vi "SetConfig.vi"(8 "error in":errorcluster, 10 "S2Config":T1 {"EC_PTEST_DELTA_BASELINE" format="%#_g psi"; "EC_PTEST_SCALE_FACTOR" min=0.0 max=1.0 step=0.01; "ECZ3_POFF_STABLE" format="%#_g sec"; "EC_PSTABLE_WAIT" format="%#_g sec"; "EC_PTEST_TIMER" format="%#_g sec"; "ECLOP_TIMER" format="%#_g sec"}, 11 "Global":T2={"Report Folder Path"=path "", "PT1_MIN"=0.0, "PT1_MAX"=0.0, "VENT_PMAX"=0.0, "LOP_TARGET"=0.0, "LOP_RAMP"=0.0, "LOP_LEAK_MAX"=0.0, "HIP_TARGET"=0.0, "HIP_RAMP"=0.0, "HIP_MIN"=0.0, "HIP_MAX"=0.0, "BLEED_TIME"=0.0, "LOP_MAX"=0.0, "LOP_MIN"=0.0, "PT131Com"="COM5", "PT231Com"="COM6", "PT331Com"="COM7", "PT431Com"="COM8", "PT531Com"="COM9", "PT631Com"="COM10"} {"LOP_MIN" format="%#_g PSI"; "LOP_MAX" format="%#_g PSI"; "BLEED_TIME" format="%#_g Sec"; "HIP_MAX" format="%#_g PSI"; "HIP_MIN" format="%#_g PSI"; "HIP_RAMP" format="%#_g Sec"; "HIP_TARGET" format="%#_g PSI"; "LOP_LEAK_MAX" format="%#_g PSI"; "LOP_RAMP" format="%#_g Sec"; "LOP_TARGET" format="%#_g PSI"; "VENT_PMAX" format="%#_g PSI"; "PT1_MAX" format="%#_g PSI"; "PT1_MIN" format="%#_g PSI"}) -> (0 "error out":errorcluster)   [LabVIEW 2018, in "S2.lvclass"]
uses:
  S2.lvclass
  Controller/Public Controls/GlobalConfig.ctl
  Controller/Public Controls/S2Config.ctl
  Queue/Queue Data.ctl
  Queue/State.ctl
  Controller/GUI.lvclass
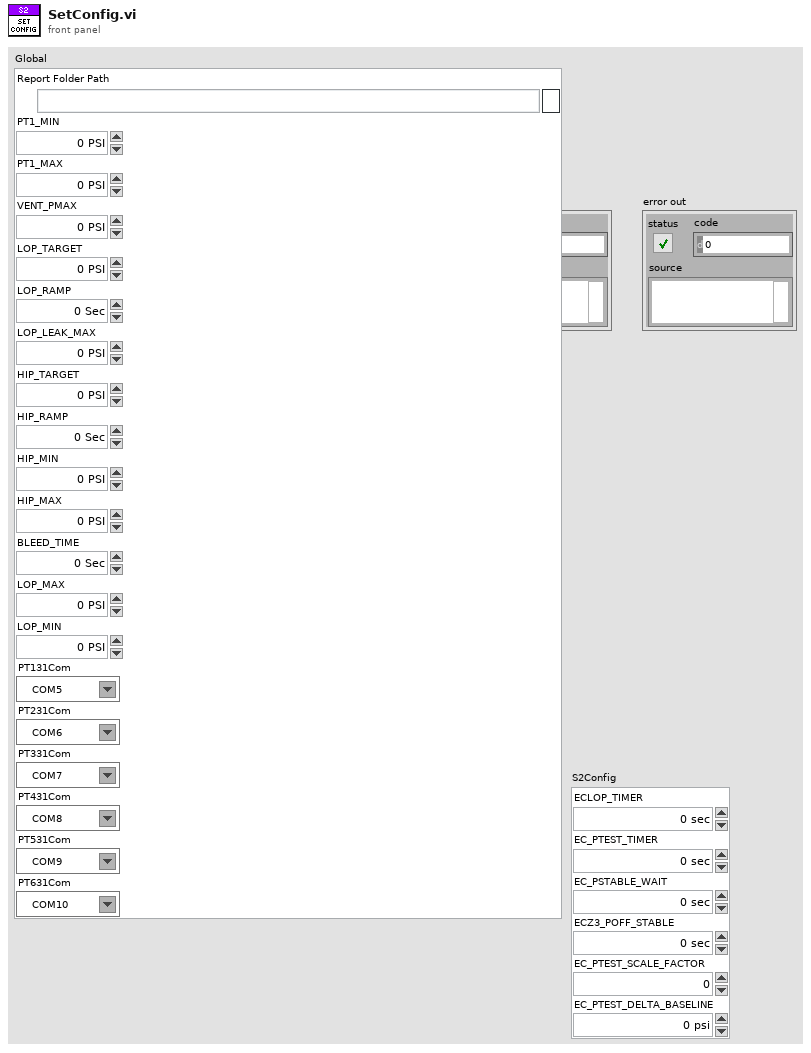
[diagram p1: front panel]
types:
  T1 = typedef "GUI.lvclass/S2Config.ctl" = cluster{"ECLOP_TIMER":dbl, "EC_PTEST_TIMER":dbl, "EC_PSTABLE_WAIT":dbl, "ECZ3_POFF_STABLE":dbl, "EC_PTEST_SCALE_FACTOR":dbl, "EC_PTEST_DELTA_BASELINE":dbl}
  T2 = typedef "GUI.lvclass/GlobalConfig.ctl" = cluster{"Report Folder Path":path, "PT1_MIN":dbl, "PT1_MAX":dbl, "VENT_PMAX":dbl, "LOP_TARGET":dbl, "LOP_RAMP":dbl, "LOP_LEAK_MAX":dbl, "HIP_TARGET":dbl, "HIP_RAMP":dbl, "HIP_MIN":dbl, "HIP_MAX":dbl, "BLEED_TIME":dbl, "LOP_MAX":dbl, "LOP_MIN":dbl, "PT131Com":refnum<visa-resource-name>, "PT231Com":refnum<visa-resource-name>, "PT331Com":refnum<visa-resource-name>, "PT431Com":refnum<visa-resource-name>, "PT531Com":refnum<visa-resource-name>, "PT631Com":refnum<visa-resource-name>}
  T3 = typedef "S2.lvclass/Queue Data.ctl" = cluster{"State":T4, "Data":variant}
  T4 = typedef "S2.lvclass/State.ctl" = enum16{"Initialize", "SetConfig", "AckAlarm", "Alarm", "Idle", "LockLid", "LowPressure", "Pressurize", "DecayTest", "Vent", "Abort", "Start", "CreateReports", "WriteToReport", "WritePressure", "Error", "Exit"}
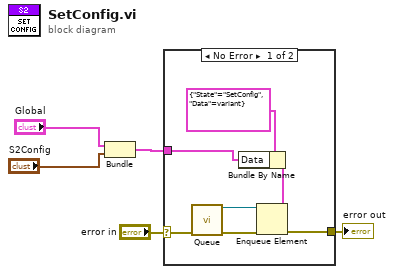
[diagram p0: block diagram]
diagram:
  n1 = Bundle("Global"="Global", "S2Config"="S2Config") -> (w1:cluster{"Global":T2, "S2Config":T1})  [unwired: 1 in]
  n2 = case shown="No Error" "error in" {
    selector: "error in" -> [w12 w13]
    tunnel: [w9 w13] -> w5
    tunnel: w1 -> [w6 _]
    frame No Error {
      n3 = call "Queue.vi"("error in"=w12) -> ("error out"=w11:errorcluster, "queue out"=w10:refnum<queue>)  [unwired: 9 in]
      n4 = Bundle By Name(cluster=T3 {"State"=enum."SetConfig", "Data"=variant} ("element"), "Data"=w6) -> (w7:T3)
      n5 = Enqueue Element(queue=w10, element=w7, error in (no error)=w11) -> (error out=w9:errorcluster)  [unwired: 1 in, 2 out]
    }
    frame Error {
    }
  }
  "error out" <- w5
